vi "Actual Record Length Core.vi"(8 "error in (no error)":errorcluster, 11 "CS++Scope":refnum<class "CS++Scope.lvclass">) -> (0 "error out":errorcluster, 2 "actual record length":i32 caption="actual record length (samples)", 3 "CS++Scope out":refnum<class "CS++Scope.lvclass">)   [LabVIEW 2015, in "CS++Scope.lvlib" / "CS++Scope.lvclass"]
doc: "This VI returns the actual number of points the oscilloscope acquires for each channel. After you configure the oscilloscope for an acquisition, call this VI to determine the size of the waveforms that the oscilloscope acquires. The value is greater than or equal to the minimum number of points you specify in the IviScope Configure Acquisition Record VI. \nYou can use this value as the Waveform Size parameter of the IviScope Read Waveform and IviScope Fetch Waveform VIs."
uses:
  CS++Scope.lvclass
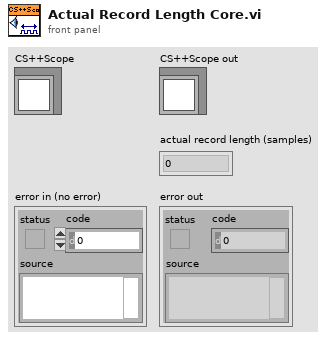
[diagram p1: front panel]
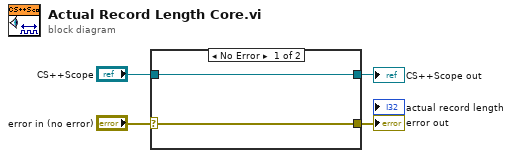
[diagram p0: block diagram]
diagram:
  n1 = case shown="No Error" "error in (no error)" {
    selector: "error in (no error)" -> [w5 w8]
    tunnel: [w5 w8] -> w3
    tunnel: [w6 w7] -> w1
    tunnel: "CS++Scope" -> [w6 w7]
    frame No Error {
    }
    frame Error {
    }
  }
  "error out" <- w3
  "CS++Scope out" <- w1
